vi "VCI_CAN_OBJ_1_CONVERT.vi"(1 "VCI_CAN_OBJ_1":T2) -> (0 "VCI_CAN_OBJ":T1)   [LabVIEW 2018, in "ControlCan.lvlib"]
uses:
  ControlCan.lvlib
  VCI_CAN_OBJ_1.ctl
  VCI_CAN_OBJ.ctl
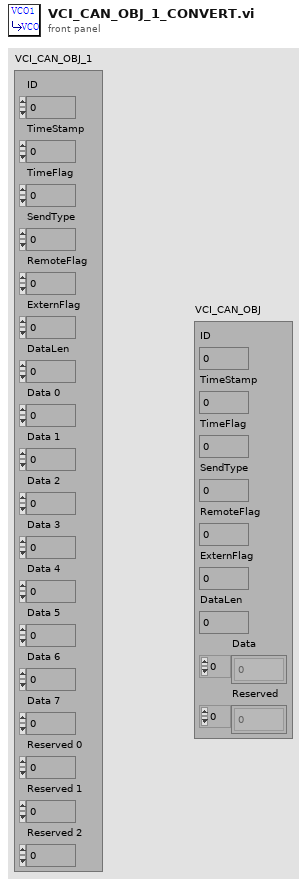
[diagram p1: front panel]
types:
  T1 = typedef "ControlCAN.lvlib/VCI_CAN_OBJ.ctl" = cluster{"ID":u32, "TimeStamp":u32, "TimeFlag":u8, "SendType":u8, "RemoteFlag":u8, "ExternFlag":u8, "DataLen":u8, "Data":u8[], "Reserved":u8[]}
  T2 = typedef "ControlCAN.lvlib/VCI_CAN_OBJ_1.ctl" = cluster{"ID":u32, "TimeStamp":u32, "TimeFlag":u8, "SendType":u8, "RemoteFlag":u8, "ExternFlag":u8, "DataLen":u8, "Data 0":u8, "Data 1":u8, "Data 2":u8, "Data 3":u8, "Data 4":u8, "Data 5":u8, "Data 6":u8, "Data 7":u8, "Reserved 0":u8, "Reserved 1":u8, "Reserved 2":u8}
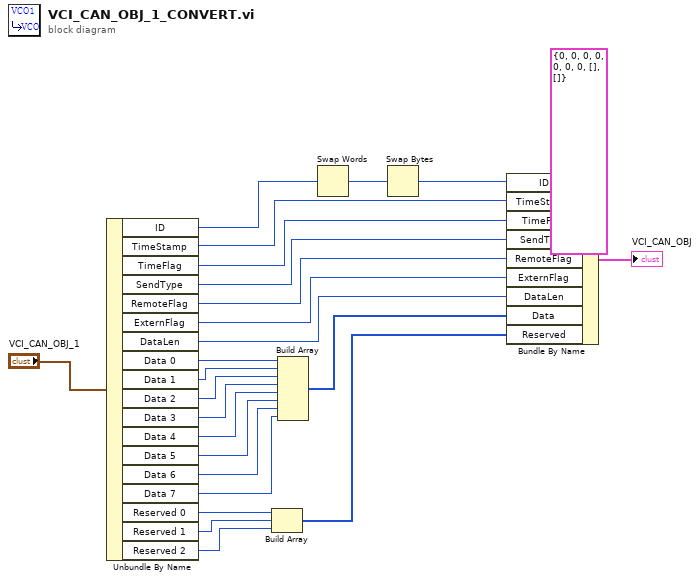
[diagram p0: block diagram]
diagram:
  n1 = Unbundle By Name("VCI_CAN_OBJ_1") -> ("ID"=w2:u32, "TimeStamp"=w23:u32, "TimeFlag"=w22:u8, "SendType"=w21:u8, "RemoteFlag"=w20:u8, "ExternFlag"=w4:u8, "DataLen"=w19:u8, "Data 0"=w18:u8, "Data 1"=w17:u8, "Data 2"=w16:u8, "Data 3"=w15:u8, "Data 4"=w14:u8, "Data 5"=w13:u8, "Data 6"=w12:u8, "Data 7"=w11:u8, "Reserved 0"=w9:u8, "Reserved 1"=w8:u8, "Reserved 2"=w7:u8)
  n2 = Build Array(w9, w8, w7) -> (w6:u8[])
  n3 = Build Array(w18, w17, w16, w15, w14, w13, w12, w11) -> (w10:u8[])
  n4 = Swap Words(1:w2) -> (0:w3:u32)
  n5 = Swap Bytes(anything=w3) -> (byte swapped=w1:u32)
  n6 = Bundle By Name(cluster=T1 {"ID"=0, "TimeStamp"=0, "TimeFlag"=0, "SendType"=0, "RemoteFlag"=0, "ExternFlag"=0, "DataLen"=0, "Data"=[], "Reserved"=[]} ("VCI_CAN_OBJ"), "ID"=w1, "TimeStamp"=w23, "TimeFlag"=w22, "SendType"=w21, "RemoteFlag"=w20, "ExternFlag"=w4, "DataLen"=w19, "Data"=w10, "Reserved"=w6) -> (→"VCI_CAN_OBJ":T1)
